vi "_moveVIToCallerCenter.vi"(8 "error in (no error)":errorcluster, 10 "CallerVI in":refnum<vi>, 11 "VI in":refnum<vi>) -> (0 "error out":errorcluster, 2 "CallerVI out":refnum<vi>, 3 "VI out":refnum<vi>)   [LabVIEW 2014, in "UI_ProgressDlg.lvlib" / "UI_ProgressDlg.lvclass"]
uses:
  UI_ProgressDlg.lvclass
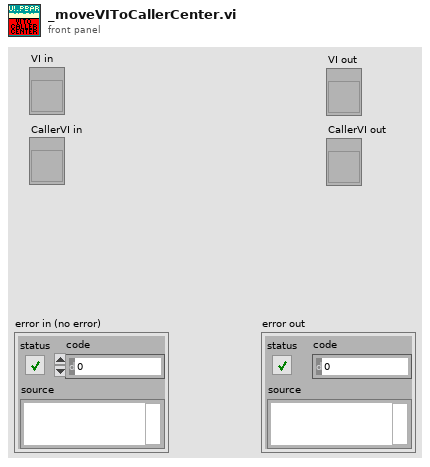
[diagram p1: front panel]
types:
  T1 = typedef "LVRectTypeDef.ctl" = cluster{"Left":i16, "Top":i16, "Right":i16, "Bottom":i16}
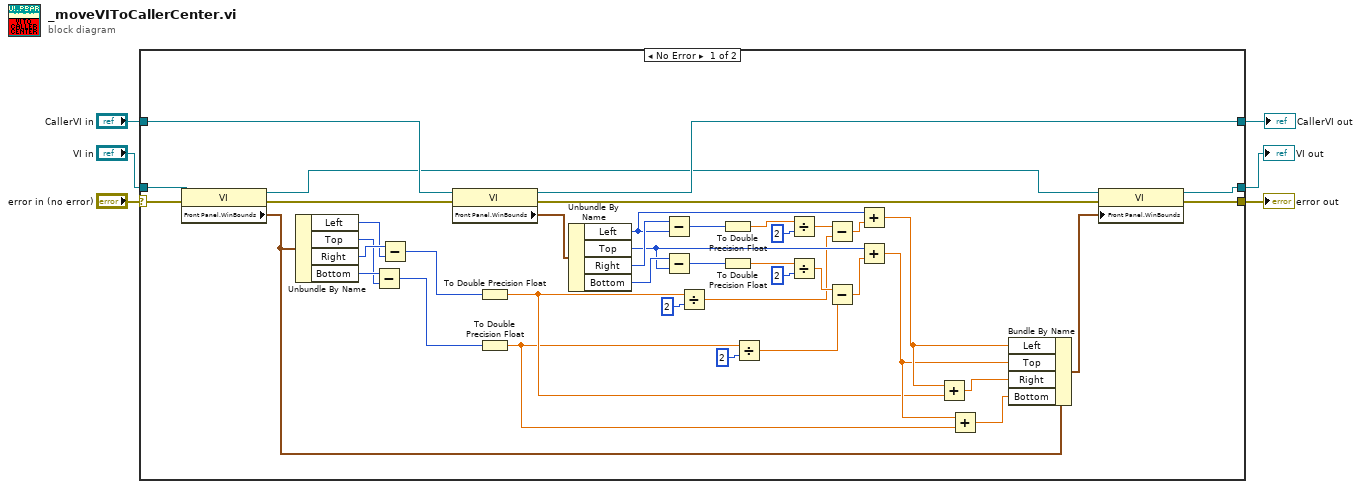
[diagram p0: block diagram]
diagram:
  n1 = case shown="No Error" "error in (no error)" {
    selector: "error in (no error)" -> [w37 w51]
    tunnel: [w48 w50] -> w6
    tunnel: "VI in" -> [w38 w50]
    tunnel: [w36 w51] -> w3
    tunnel: "CallerVI in" -> [w25 w49]
    tunnel: [w24 w49] -> w1
    frame No Error {
      n2 = property on="Property Node" class="VI"(reference=w38, error in=w37) -> (reference out=w9:refnum<vi>, error out=w44:errorcluster, "Front Panel.WinBounds"=w17:T1)
      n3 = Unbundle By Name(w17) -> ("Left"=w20:i16, "Top"=w21:i16, "Right"=w22:i16, "Bottom"=w23:i16)
      n4 = Subtract(x=w23, y=w21) -> (x-y=w18:i16)
      n5 = Subtract(x=w22, y=w20) -> (x-y=w19:i16)
      n6 = property class="VI"(reference=w25, error in=w44) -> (reference out=w24:refnum<vi>, error out=w45:errorcluster, "Front Panel.WinBounds"=w43:T1)
      n7 = To Double Precision Float(number=w19) -> (double precision float=w13:dbl)
      n8 = To Double Precision Float(number=w18) -> (double precision float=w12:dbl)
      n9 = Unbundle By Name(w43) -> ("Left"=w29:i16, "Top"=w28:i16, "Right"=w32:i16, "Bottom"=w31:i16)
      n10 = Subtract(x=w32, y=w29) -> (x-y=w33:i16)
      n11 = Subtract(x=w31, y=w28) -> (x-y=w30:i16)
      n12 = Divide(x=w13, y=u32 2) -> (x/y=w8:dbl)
      n13 = To Double Precision Float(number=w33) -> (double precision float=w27:dbl)
      n14 = To Double Precision Float(number=w30) -> (double precision float=w26:dbl)
      n15 = Divide(x=w12, y=u32 2) -> (x/y=w7:dbl)
      n16 = Divide(x=w27, y=u32 2) -> (x/y=w34:dbl)
      n17 = Divide(x=w26, y=u32 2) -> (x/y=w35:dbl)
      n18 = Subtract(x=w34, y=w8) -> (x-y=w46:dbl)
      n19 = Subtract(x=w35, y=w7) -> (x-y=w47:dbl)
      n20 = Add(x=w29, y=w46) -> (x+y=w15:dbl)
      n21 = Add(x=w28, y=w47) -> (x+y=w14:dbl)
      n22 = Add(x=w15, y=w13) -> (x+y=w11:dbl)
      n23 = Add(x=w14, y=w12) -> (x+y=w10:dbl)
      n24 = Bundle By Name(cluster=w17, "Left"=w15, "Top"=w14, "Right"=w11, "Bottom"=w10) -> (w16:T1)
      n25 = property on="Property Node" class="VI"(reference=w9, error in=w45, "Front Panel.WinBounds"=w16) -> (reference out=w48:refnum<vi>, error out=w36:errorcluster)
    }
    frame Error {
    }
  }
  "VI out" <- w6
  "error out" <- w3
  "CallerVI out" <- w1
